vi "Pockels Cal-Modify cursor index values.vi"(8 "error in (no error)":errorcluster, 10 "Single Cal table (Final format)":string[][](array[string])=[["Cal Wavelength", "", "", "", "", ""], ["920", "", "", "", "", ""], ["Cal subset indexes", "", "", "", "", ""], ["0", "15", "", "", "", ""], ["Cal data", "", "", "", "", ""], ["Pockels V", "No objective", "Olympus 20X", "Nikon 25X", "Olympus 40X", "Olympus 60X"], ["0", "0", "", "", "", ""], ["0.1", "6", "", "", "", ""], ["0.2", "10.8", "", "", "", ""], ["0.3", "16.6", "", "", "", ""], ["0.4", "23.4", "", "", "", ""], ["0.5", "30.7", "", "", "", ""], ["0.6", "38.8", "", "", "", ""], ["0.7", "46.8", "", "", "", ""], ["0.8", "54.8", "", "", "", ""], ["0.9", "62.4", "", "", "", ""], ["1", "69.4", "", "", "", ""], ["1.1", "75.3", "", "", "", ""], ["1.2", "80.3", "", "", "", ""], ["1.3", "84", "", "", "", ""], ["1.4", "86.3", "", "", "", ""], ["1.5", "87", "86.4", "", "", ""], ["1.6", "86.1", "", "", "", ""], ["1.7", "84.5", "", "", "", ""], ["1.8", "84.4", "", "", "", ""], ["1.9", "84.2", "", "", "", ""], ["2", "84.1", "", "", "", ""]], 11 "XYGraph in":refnum<vi>) -> (0 "error out":errorcluster, 2 "Single Cal table (Final format)":string[][](array[string]), 3 "XYGraph":refnum<vi>)   [LabVIEW 2013]
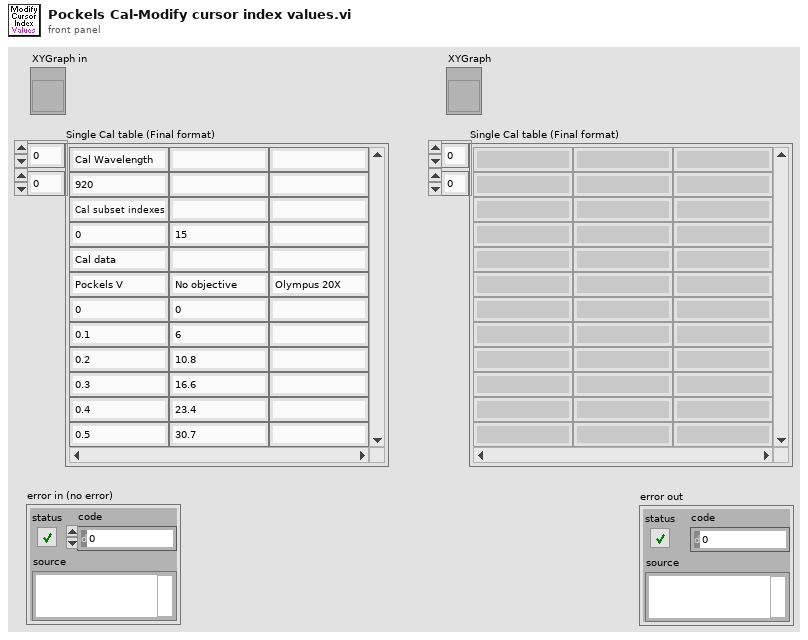
[diagram p1: front panel]
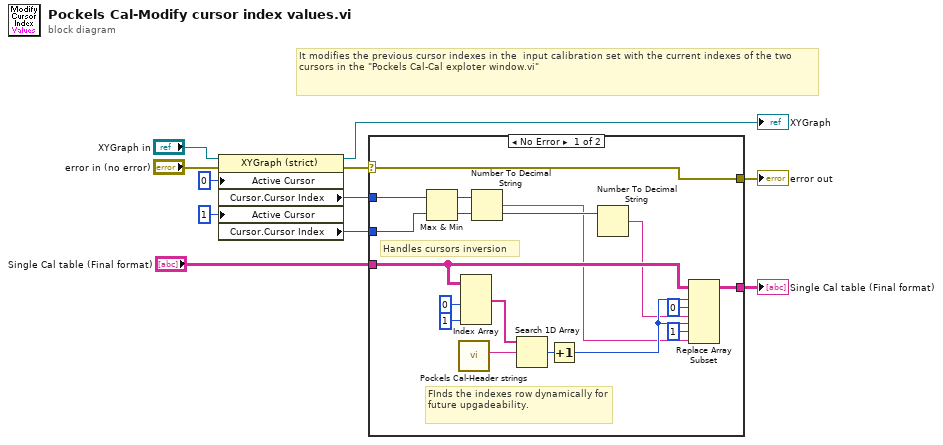
[diagram p0: block diagram]
diagram:
  # "It modifies the previous cursor indexes in the  input calibration set with the current indexes of the two cursors in the \"Pockels Cal-Cal exploter window.vi\""
  n1 = property on="Property Node" class="XYGraph (strict)"(reference="XYGraph in", error in="error in (no error)", "Active Cursor"=u32 0, "Active Cursor"=u32 1) -> (reference out=→"XYGraph":refnum<vi>, error out=w3:errorcluster, "Cursor.Cursor Index"=w9:i32, "Cursor.Cursor Index"=w8:i32)
  n2 = case shown="No Error" w3 {
    selector: w3 -> [w13 w30]
    tunnel: w9 -> [w28 _]
    tunnel: w8 -> [w27 _]
    tunnel: "Single Cal table (Final format)" -> [w20 w29]
    tunnel: [w13 w30] -> w2
    tunnel: [w14 w29] -> w1
    frame No Error {
      # "Handles cursors inversion"
      # "FInds the indexes row dynamically for future upgadeability."
      n3 = Max & Min(x=w28, y=w27) -> (max(x,y)=w25:i32, min(x,y)=w26:i32)
      n4 = call "Pockels Cal-Header strings.vi"() -> ("Cal subset indexes header string"=w12:string)  [unwired: 9 in, 2 out]
      n5 = Index Array(array=w20, index (col) #1=0 ("disabled index (col)"), index (col) #2=1 ("index (col)")) -> (element #1=w22:string[])  [unwired: 2 in, 1 out]
      n6 = Number To Decimal String(number=w25) -> (decimal integer string=w15:string)  [unwired: 1 in]
      n7 = Search 1D Array(1D array=w22, element=w12) -> (index of element=w23:i32)  [unwired: 1 in]
      n8 = Increment(x=w23) -> (x+1=w17:i32)
      n9 = Number To Decimal String(number=w26) -> (decimal integer string=w16:string)  [unwired: 1 in]
      n10 = Replace Array Subset(array=w20, new element #1=w16, index (row) #1=w17, index (col) #1=0 ("disabled index (col)"), new element #2=w15, index (row) #2=w17, index (col) #2=1 ("index (col)")) -> (w14:string[][])
    }
    frame Error {
    }
  }
  "Single Cal table (Final format)" <- w1
  "error out" <- w2
